vi "Process Collisions.vi"(11 "Laser in":refnum<class "Laser.lvclass">) -> (3 "Laser out":refnum<class "Laser.lvclass">)   [LabVIEW 2021, in "Laser.lvclass"]
uses:
  Laser.lvclass
  C:/dev/LabVIEW/LabMelee/Source/Application Specific/Element/Element.lvclass
  Element/Element.lvclass/Element.ctl
  Laser.lvclass/Laser.ctl
  Re-use Libraries/Vector 2D/Vector 2D.lvclass
  Ship/Ship.lvclass
  Motion/Motion.lvclass/Motion.ctl
  Ship/Ship.lvclass/Ship.ctl
  Element/Element.lvclass
  Re-use Libraries/Collision/Collision.lvlib
  Re-use Libraries/Utility/Typedef/Line.ctl
  Re-use Libraries/Utility/Utility.lvlib
  Resource Manager/Resource Manager.lvclass
  Globals.vi
  Motion/Motion.lvclass
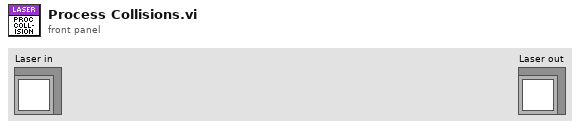
[diagram p1: front panel]
types:
  T1 = typedef "Element.lvclass/Player Type.ctl" = enum16{"Neutral", "Player 1", "Player 2"}
  T2 = typedef "Utility.lvlib/Line.ctl" = cluster{"Start Point":refnum<class "Vector 2D.lvclass">, "End Point":refnum<class "Vector 2D.lvclass">}
  T3 = typedef "Utility.lvlib/Axis Aligned Bounding Box.ctl" = cluster{"Top Left":refnum<class "Vector 2D.lvclass">, "Bottom Right":refnum<class "Vector 2D.lvclass">}
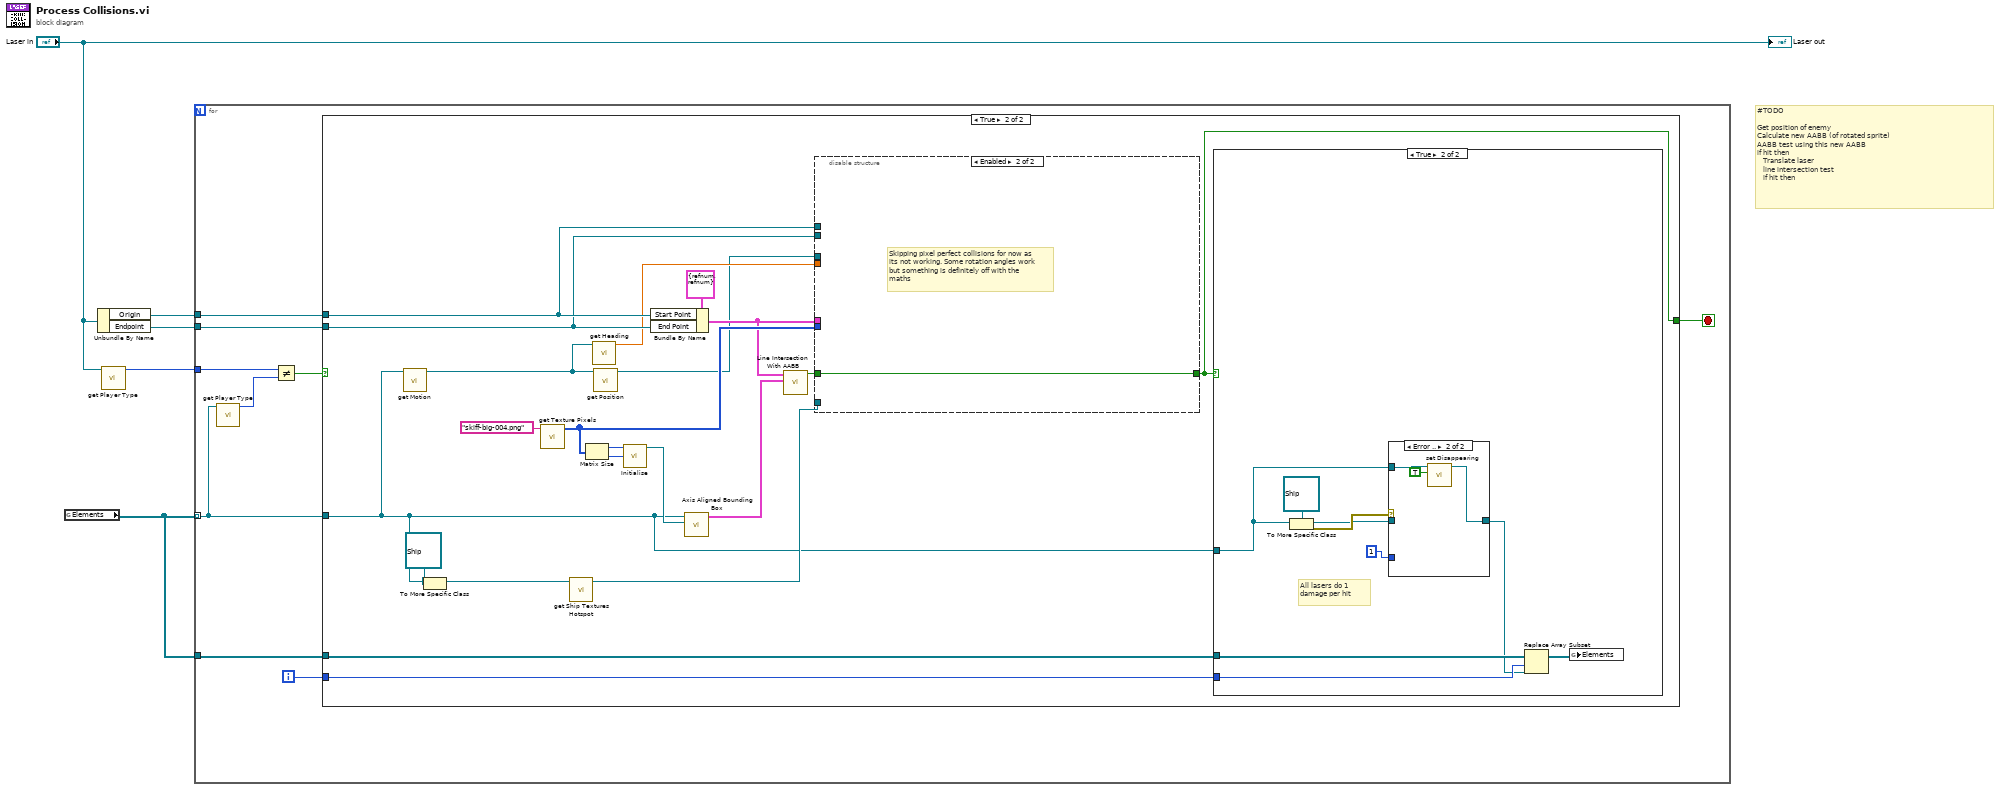
[diagram p0: block diagram]
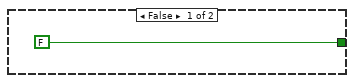
[diagram p2: hidden frame]
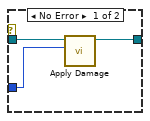
[diagram p4: hidden frame]
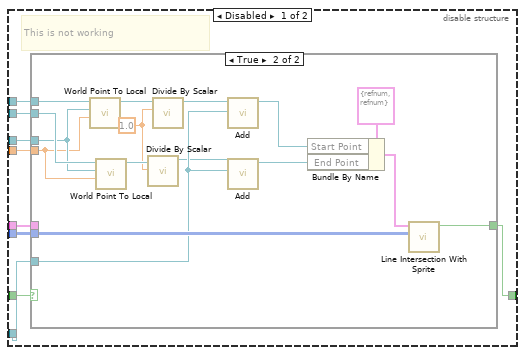
[diagram p5: hidden frame]
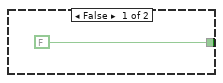
[diagram p6: hidden frame]
diagram:
  # "#TODO\n\nGet position of enemy\nCalculate new AABB (of rotated sprite)\nAABB test using this new AABB\nif hit then\n   Translate laser\n   line intersection test\n   if hit then"
  n1 = global read "Globals.vi" "Elements"() -> (w3:refnum<class "Element.lvclass">[])
  n2 = Unbundle By Name("Laser in") -> ("Origin"=w5:refnum<class "Vector 2D.lvclass">, "Endpoint"=w4:refnum<class "Vector 2D.lvclass">)
  n3 = call "get Player Type.vi"("Element in"="Laser in") -> ("Player Type"=w2:T1)  [unwired: 10 in]
  n4 = for {
    tunnel: w5 -> [w14]
    tunnel: w4 -> [w13]
    tunnel: w3 -> [w7] mode=indexing
    tunnel: w3 -> [w12]
    tunnel: w2 -> [w11]
    i -> [w6]
    stop <- w8 stop-if-true
    n5 = call "get Player Type.vi"("Element in"=w7) -> ("Player Type"=w10:T1)  [unwired: 10 in]
    n6 = Not Equal?(x=w11, y=w10) -> (x != y?=w9:bool)
    n7 = case shown="True" w9 {
      tunnel: w14 -> [_ w36]
      tunnel: w13 -> [_ w35]
      tunnel: [FALSE ("Intersects?") w16] -> w8
      tunnel: w12 -> [_ w19]
      tunnel: w7 -> [_ w17]
      tunnel: w6 -> [_ w18]
      frame False {
      }
      frame True {
        n8 = call "get Motion.vi"("Element in"=w17) -> ("Motion"=w24:refnum<class "Motion.lvclass">)  [unwired: 10 in]
        n9 = To More Specific Class(target class=refnum<class "Ship.lvclass"> refnum ("Ship.lvclass"), reference=w17) -> (specific class reference=w22:refnum<class "Ship.lvclass">)  [unwired: 1 in, 1 out]
        n10 = call "get Texture Pixels.vi"("Texture Name"="skiff-big-004.png") -> ("Pixels"=w32:u32[][])  [unwired: 10 in]
        n11 = call "get Ship Textures Hotspot.vi"("Ship in"=w22) -> ("Ship Hotspot"=w20:refnum<class "Vector 2D.lvclass">)  [unwired: 10 in]
        n12 = Matrix Size(0:w32) -> (1:w31:i32, 2:w30:i32)
        n13 = call "get Heading.vi"("Motion in"=w24) -> ("Heading [deg]"=w25:sgl)  [unwired: 10 in]
        n14 = call "get Position.vi"("Motion in"=w24) -> ("Displacement"=w21:refnum<class "Vector 2D.lvclass">)  [unwired: 10 in]
        n15 = call "Initialise.vi"("y"=w30, "x"=w31) -> ("Vector 2D out"=w29:refnum<class "Vector 2D.lvclass">)  [unwired: 9 in]
        n16 = Bundle By Name(cluster=T2 {"Start Point"=refnum, "End Point"=refnum} ("Line"), "Start Point"=w36, "End Point"=w35) -> (w28:T2)
        n17 = call "Axis Aligned Bounding Box.vi"("Texture Size"=w29, "Element in"=w17) -> ("AABB"=w27:T3)  [unwired: 9 in]
        n18 = call "Line Intersection With AABB.vi"("AABB"=w27, "Line"=w28) -> ("Intersects?"=w26:bool)  [unwired: 9 in]
        n19 = disable-structure shown="Enabled" {
          disable-tunnel: w32 -> [w60 _]
          disable-tunnel: w28 -> [w59 _]
          disable-tunnel: w26 -> [w58 w78]
          disable-tunnel: w36 -> [w57 _]
          disable-tunnel: w35 -> [w56 _]
          disable-tunnel: w25 -> [w55 _]
          disable-tunnel: [w54 w78] -> w16
          disable-tunnel: w21 -> [w53 _]
          disable-tunnel: w20 -> [w52 _]
          frame Disabled {
            # "This is not working"
            n20 = case shown="True" w58 {
              tunnel: w60 -> [_ w77]
              tunnel: w59 -> [_ _]
              tunnel: w57 -> [_ w76]
              tunnel: w56 -> [_ w75]
              tunnel: w53 -> [_ w74]
              tunnel: w55 -> [_ w73]
              tunnel: [FALSE ("Hit") w70] -> w54
              tunnel: w52 -> [_ w68]
              frame False {
              }
              frame True {
                w63 = sgl 1.0 ("x")
                n21 = call "World Point To Local.vi"("Rotation [deg]"=w73, "Sprite Center"=w74, "World Point"=w76) -> ("Local Point"=w66:refnum<class "Vector 2D.lvclass">)  [unwired: 8 in]
                n22 = call "World Point To Local.vi"("Rotation [deg]"=w73, "Sprite Center"=w74, "World Point"=w75) -> ("Local Point"=w64:refnum<class "Vector 2D.lvclass">)  [unwired: 8 in]
                n23 = call "Divide By Scalar.vi"("x"=w63, "A"=w64) -> ("Ax"=w62:refnum<class "Vector 2D.lvclass">)  [unwired: 9 in]
                n24 = call "Divide By Scalar.vi"("x"=w63, "A"=w66) -> ("Ax"=w65:refnum<class "Vector 2D.lvclass">)  [unwired: 9 in]
                n25 = call "Add.vi"("B"=w68, "A"=w65) -> ("A+B"=w69:refnum<class "Vector 2D.lvclass">)  [unwired: 9 in]
                n26 = call "Add.vi"("B"=w68, "A"=w62) -> ("A+B"=w67:refnum<class "Vector 2D.lvclass">)  [unwired: 9 in]
                n27 = Bundle By Name(cluster=T2 {"Start Point"=refnum, "End Point"=refnum} ("Line"), "Start Point"=w69, "End Point"=w67) -> (w71:T2)
                n28 = call "Line Intersection With Sprite.vi"("Pixel Data in"=w77, "Line"=w71) -> ("Hit"=w70:bool)  [unwired: 8 in, 1 out]
              }
            }
          }
          frame Enabled {
            # "Skipping pixel perfect collisions for now as its not working. Some rotation angles work but something is definitely off with the maths"
          }
        }
        n29 = case shown="True" w16 {
          tunnel: w19 -> [_ w44]
          tunnel: w18 -> [_ w43]
          tunnel: w17 -> [_ w38]
          frame False {
          }
          frame True {
            # "All lasers do 1 damage per hit"
            n30 = To More Specific Class(target class=refnum<class "Ship.lvclass"> refnum ("Ship in"), reference=w38) -> (specific class reference=w40:refnum<class "Ship.lvclass">, error out=w41:errorcluster)  [unwired: 1 in]
            n31 = case shown="Error .." w41 {
              tunnel: w40 -> [w48 _]
              tunnel: [w47 w50] -> w39
              tunnel: w38 -> [_ w51]
              tunnel: 1 ("Damage") -> [w46 _]
              frame No Error {
                n32 = call "Apply Damage.vi"("Damage"=w46, "Ship in"=w48) -> ("Ship out"=w47:refnum<class "Ship.lvclass">)  [unwired: 9 in]
              }
              frame Error {
                n33 = call "set Disappearing.vi"("Disappearing"=TRUE, "Element in"=w51) -> ("Element out"=w50:refnum<class "Element.lvclass">)  [unwired: 9 in]
              }
            }
            n34 = Replace Array Subset(array=w44, new element=w39, index=w43) -> (w45:refnum<class "Element.lvclass">[])
            n35 = global write "Globals.vi" "Elements"(w45) -> ()
          }
        }
      }
    }
  }
  "Laser out" <- "Laser in"
